vi "configure.vi"(7 "Save Data":bool=TRUE, 8 "error in (no error)":errorcluster, 11 "QuadraturePositionDecoder in":refnum<class "QuadraturePositionDecoder.lvclass">) -> (0 "error out":errorcluster, 3 "QuadraturePositionDecoder out":refnum<class "QuadraturePositionDecoder.lvclass">)   [LabVIEW 2014, in "QuadraturePositionDecoder.lvclass"]
uses:
  QuadraturePositionDecoder.lvclass
  QuadraturePositionDecoder.lvclass/QuadraturePositionDecoder.ctl
  <vilib>/DAQmx/create/channels.llb/DAQmx Create Channel (CI-Position-Angular Encoder).vi
  <resource>/objmgr/daqmx.rc
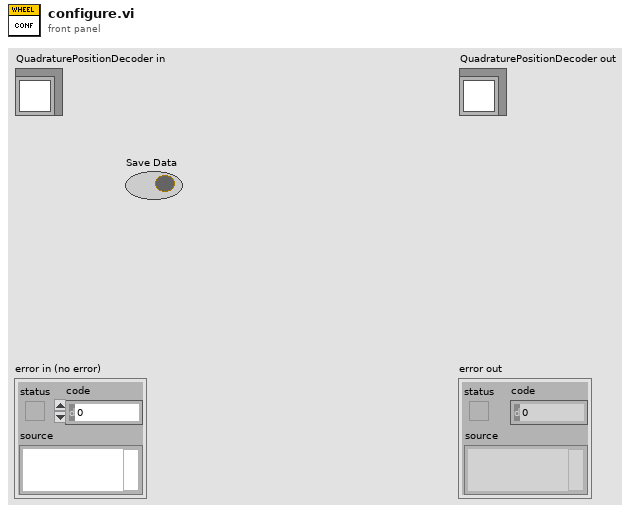
[diagram p1: front panel]
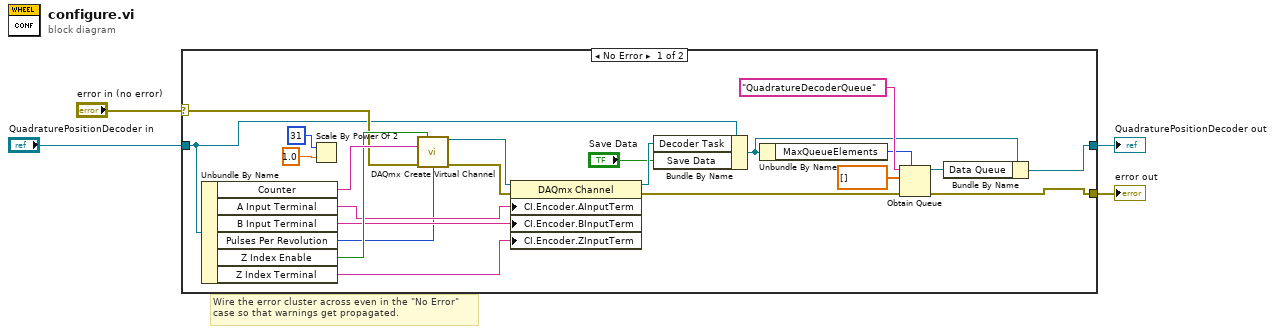
[diagram p0: block diagram]
diagram:
  # "Wire the error cluster across even in the \"No Error\"\ncase so that warnings get propagated."
  n1 = case shown="No Error" "error in (no error)" {
    selector: "error in (no error)" -> [w20 w28]
    tunnel: [w5 w28] -> w3
    tunnel: "QuadraturePositionDecoder in" -> [w7 w27]
    tunnel: [w6 w27] -> w1
    frame No Error {
      n2 = Unbundle By Name(w7) -> ("Counter"=w25:tag, "A Input Terminal"=w23:tag, "B Input Terminal"=w22:tag, "Pulses Per Revolution"=w8:u32, "Z Index Enable"=w24:bool, "Z Index Terminal"=w21:tag)
      n3 = Scale By Power Of 2(n=i16 31, x=1.0) -> ()  [unwired: 1 out]
      n4 = call-poly <vilib>:"DAQmx Create Virtual Channel.vi"("z index enable"=w24, "counter"=w25, "error in"=w20, "pulses per revolution"=w8) -> ("task out"=w26:refnum<k21>, "error out"=w19:errorcluster)  [unwired: 10 in]
      n5 = property class="DAQmx Channel"(reference=w26, error in=w19, "CI.Encoder.AInputTerm"=w23, "CI.Encoder.BInputTerm"=w22, "CI.Encoder.ZInputTerm"=w21) -> (reference out=w18:refnum<k21>, error out=w14:errorcluster)
      n6 = Bundle By Name(cluster=w7, "Decoder Task"=w18, "Save Data"="Save Data") -> (w13:refnum<class "QuadraturePositionDecoder.lvclass">)
      n7 = Unbundle By Name(w13) -> ("MaxQueueElements"=w12:i32)
      n8 = Obtain Queue(max queue size (-1, unlimited)=w12, name (unnamed)="QuadratureDecoderQueue", element data type=dbl[] [] ("appended array"), error in (no error)=w14) -> (queue out=w15:refnum<queue>, error out=w5:errorcluster)  [unwired: 1 in, 1 out]
      n9 = Bundle By Name(cluster=w13, "Data Queue"=w15) -> (w6:refnum<class "QuadraturePositionDecoder.lvclass">)
    }
    frame Error {
    }
  }
  "error out" <- w3
  "QuadraturePositionDecoder out" <- w1
